vi "Get Sweep.vi"(0 "Sweep Name":string, 11 "error in (no error)":errorcluster) -> (4 "Sweep":T1, 6 "Sweep not found?":bool, 15 "error out":errorcluster)   [LabVIEW 2023, in "RFFixtureCharact.Public.lvlib" / "Scalar Path.lvclass"]
uses:
  Scalar Path.lvclass
  Scalar Path Group/Type Definitions/Sweep.ctl
  Common/RFCalAndFixtureCharact.Common.lvlib
  Scalar Path Group/Scalar Path Group.lvclass
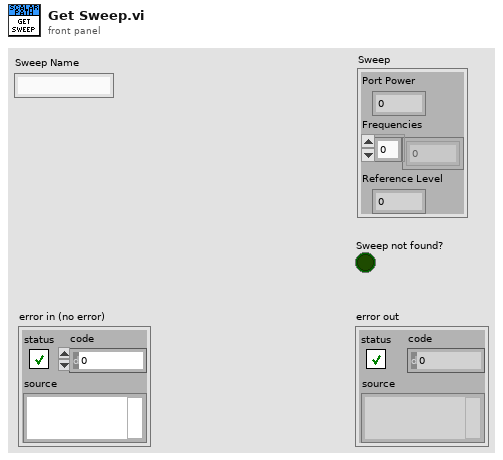
[diagram p1: front panel]
types:
  T1 = typedef "RFFixtureCharact.Public.lvlib/Scalar Path Group.lvclass/Sweep.ctl" = cluster{"Port Power":dbl, "Frequencies":dbl[], "Reference Level":dbl}
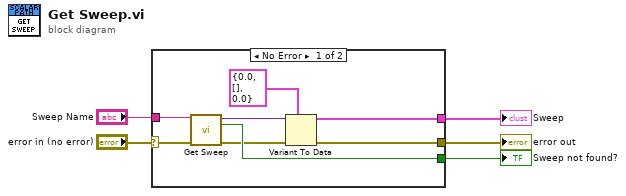
[diagram p0: block diagram]
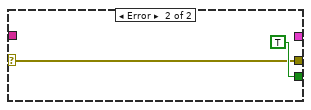
[diagram p2: hidden frame]
diagram:
  n1 = case shown="No Error" "error in (no error)" {
    selector: "error in (no error)" -> [w8 w14]
    tunnel: "Sweep Name" -> [w13 _]
    tunnel: [w6 w14] -> w4
    tunnel: [w12 TRUE ("Sweep not found?")] -> w3
    tunnel: [w9 _] -> w2
    frame No Error {
      n2 = call "Get Sweep.vi"("Sweep Name"=w13, "error in (no error)"=w8) -> ("Variant"=w11:variant, "Sweep not found?"=w12:bool, "error out"=w7:errorcluster)  [unwired: 11 in]
      n3 = Variant To Data(error in=w7, type=T1 {"Port Power"=0.0, "Frequencies"=[], "Reference Level"=0.0} ("Sweep"), Variant=w11) -> (data=w9:T1, error out=w6:errorcluster)
    }
    frame Error {
    }
  }
  "error out" <- w4
  "Sweep not found?" <- w3
  "Sweep" <- w2
